vi "MP_Generator.vi"(3 "Time Resolution (ms)":dbl, 4 "Goal (deg)":dbl, 5 "Maximum Acceleration (deg/s^2)":dbl, 6 "Maximum Velocity (deg/s)":dbl) -> (0 "Total Profile Time (s)":dbl, 1 "Timestamp (s)":dbl[](array[numeric]), 2 "Velocity (deg/s)":dbl[](array[numeric]))   [LabVIEW 2020]
panel:
  in  "Decel Index":dbl=100000000000000.0
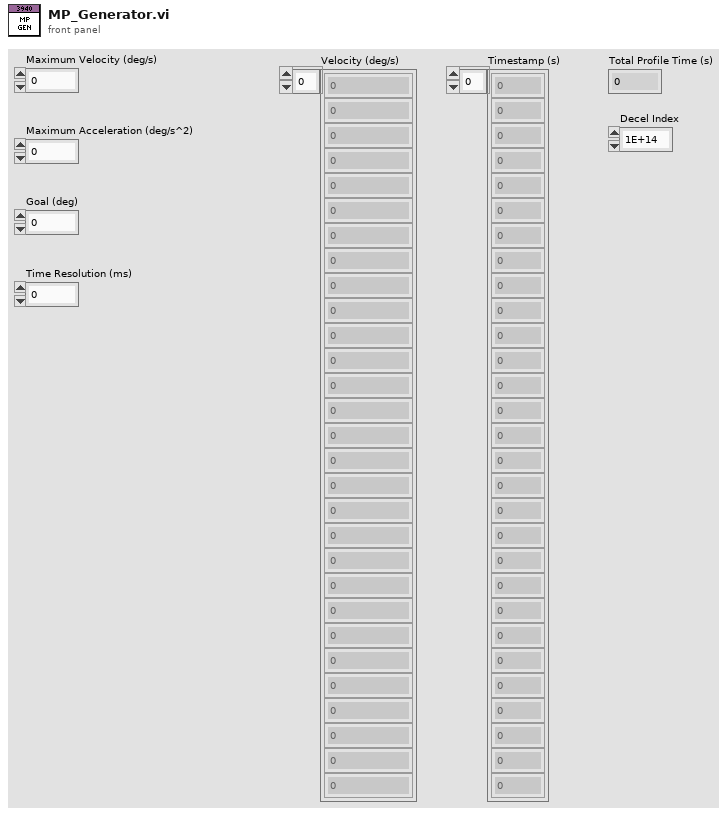
[diagram p1: front panel]
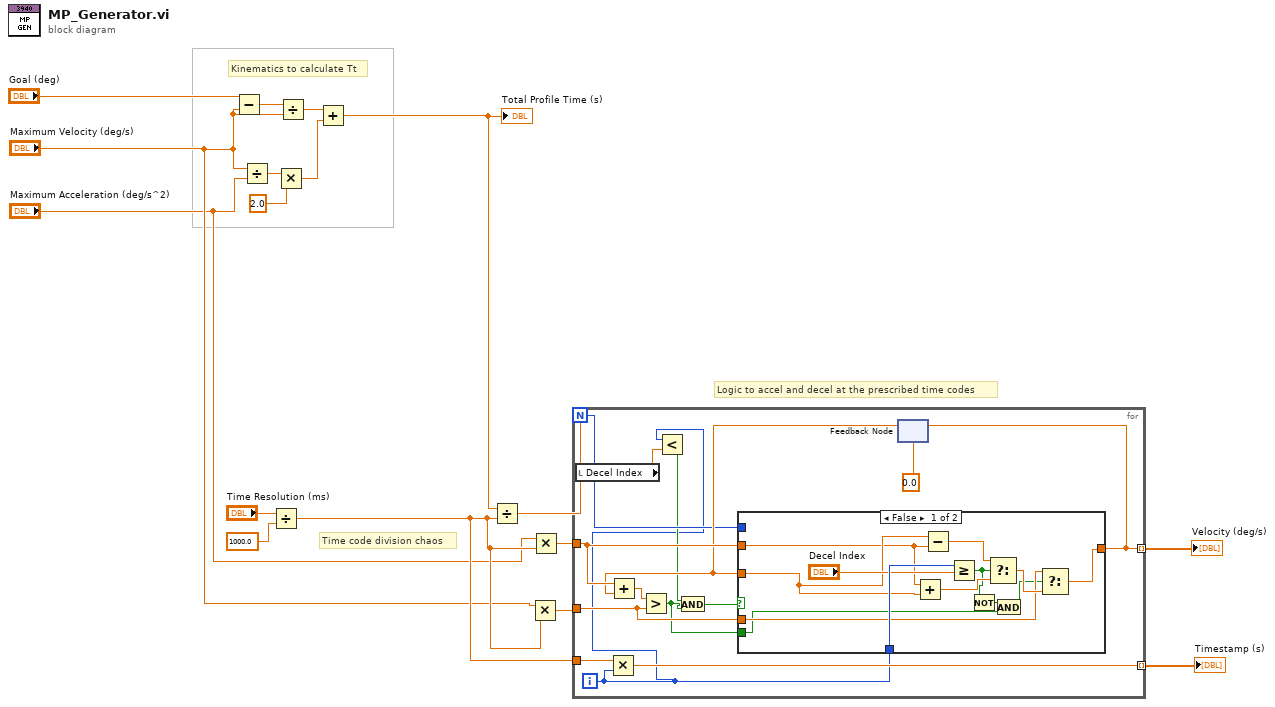
[diagram p0: block diagram]
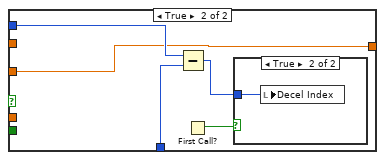
[diagram p2: hidden frame]
diagram:
  # "Time code division chaos"
  # "Logic to accel and decel at the prescribed time codes"
  # "Kinematics to calculate Tt"
  n1 = Subtract(x="Goal (deg)", y="Maximum Velocity (deg/s)") -> (x-y=w8:dbl)
  n2 = Divide(x="Maximum Velocity (deg/s)", y="Maximum Acceleration (deg/s^2)") -> (x/y=w4:dbl)
  n3 = Divide(x="Time Resolution (ms)", y=1000.0) -> (x/y=w10:dbl)
  n4 = Multiply(x=w4, y=2.0) -> (x*y=w2:dbl)
  n5 = Divide(x=w8, y="Maximum Velocity (deg/s)") -> (x/y=w7:dbl)
  n6 = Add(x=w7, y=w2) -> (x+y=w1:dbl)
  "Total Profile Time (s)" <- w1
  n7 = Divide(x=w1, y=w10) -> (x/y=w15:dbl)
  n8 = Multiply(x="Maximum Velocity (deg/s)", y=w10) -> (x*y=w11:dbl)
  n9 = Multiply(x="Maximum Acceleration (deg/s^2)", y=w10) -> (x*y=w14:dbl)
  n10 = for {
    N: w15 -> [w23]
    tunnel: w14 -> [w28]
    tunnel: [w25] -> w13 mode=indexing
    tunnel: w10 -> [w31]
    tunnel: [w30] -> w12 mode=indexing
    tunnel: w11 -> [w20]
    i -> [w18]
    n11 = local read "Decel Index"() -> (w22:dbl)
    n12 = Multiply(x=w31, y=w18) -> (x*y=w30:dbl)
    n13 = Less?(x=w18, y=w22) -> (x < y?=w21:bool)
    n14 = feedback #1(0.0) -> (w26:dbl)
    n15 = Add(x=w28, y=w26) -> (x+y=w29:dbl)
    n16 = Greater?(x=w29, y=w20) -> (0:w19:bool)
    n17 = And(x=w21, y=w19) -> (x .and. y?=w24:bool)
    n18 = case shown="False" w24 {
      tunnel: [w38 w47] -> w25
      tunnel: w18 -> [w44 w48]
      tunnel: w23 -> [_ w49]
      tunnel: w28 -> [w39 _]
      tunnel: w26 -> [w40 w47]
      tunnel: w20 -> [w36 _]
      tunnel: w19 -> [w34 _]
      frame False {
        n19 = Add(x=w39, y=w40) -> (x+y=w42:dbl)
        n20 = Subtract(x=w40, y=w39) -> (x-y=w41:dbl)
        n21 = Greater Or Equal?(x=w44, y="Decel Index") -> (x >= y?=w32:bool)
        n22 = Not(x=w32) -> (.not. x?=w33:bool)
        n23 = Select(t=w41, s=w32, f=w42) -> (s? t:f=w37:dbl)
        n24 = And(x=w33, y=w34) -> (x .and. y?=w35:bool)
        n25 = Select(t=w36, s=w35, f=w37) -> (s? t:f=w38:dbl)
      }
      frame True {
        n26 = Subtract(x=w49, y=w48) -> (x-y=w45:i32)
        n27 = First Call?() -> (First Call?: T/F=w46:bool)
        n28 = case shown="True" w46 {
          tunnel: w45 -> [_ w50]
          frame False {
          }
          frame True {
            n29 = local write "Decel Index"(w50) -> ()
          }
        }
      }
    }
    n30 = feedback-in #1(w25) -> ()
  }
  "Velocity (deg/s)" <- w13
  "Timestamp (s)" <- w12
